vi "Enqueue - Multiple Commands.vi"(5 "Insert? (T)":bool=TRUE, 7 "At Front?":bool, 8 "error in":errorcluster, 10 "Array of Commands":string[](array[string]), 11 "Queue with Cluster Reference":T1) -> (0 "error out":errorcluster, 3 "Queue (dup)":T1)   [LabVIEW 2010]
uses:
  TYP_Queue with Cluster Reference.ctl
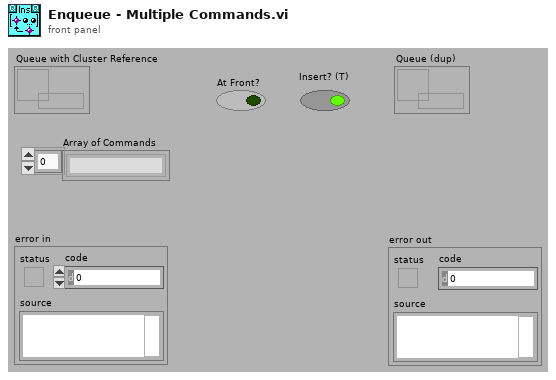
[diagram p1: front panel]
types:
  T1 = typedef "TYP_Queue with Cluster Reference.ctl" = refnum<queue>
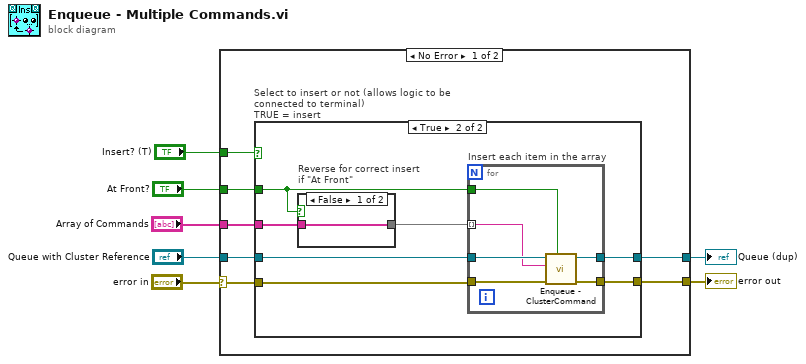
[diagram p0: block diagram]
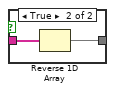
[diagram p3: hidden frame]
diagram:
  n1 = case shown="No Error" "error in" {
    selector: "error in" -> [w10 w34]
    tunnel: "Array of Commands" -> [w14 _]
    tunnel: "Queue with Cluster Reference" -> [w13 w33]
    tunnel: [w12 w33] -> w3
    tunnel: [w11 w34] -> w6
    tunnel: "At Front?" -> [w9 _]
    tunnel: "Insert? (T)" -> [w8 _]
    frame No Error {
      n2 = case "Select to insert or not (allows logic to be connected to terminal)\nTRUE = insert" shown="True" w8 {
        tunnel: w14 -> [_ w19]
        tunnel: w13 -> [w16 w23]
        tunnel: [w16 w22] -> w12
        tunnel: [w15 w21] -> w11
        tunnel: w10 -> [w15 w20]
        tunnel: w9 -> [_ w18]
        frame False {
        }
        frame True {
          n3 = case "Reverse for correct insert\nif \"At Front\"" shown="False" w18 {
            tunnel: w19 -> [w24 w26]
            tunnel: [w24 w25] -> w17
            frame False {
            }
            frame True {
              n4 = Reverse 1D Array(array=w26) -> (reversed array=w25:string[])
            }
          }
          n5 = for "Insert each item in the array" {
            tunnel: w23 -> [w29]
            tunnel: w20 -> [w32]
            tunnel: [w30] -> w22
            tunnel: [w31] -> w21
            tunnel: w17 -> [w28] mode=indexing
            tunnel: w18 -> [w27]
            n6 = call "Enqueue - ClusterCommand.vi"("At Front?"=w27, "error in (no error)"=w32, "Command"=w28, "Queue with Cluster Reference"=w29) -> ("error out"=w31:errorcluster, "Queue Out (dup)"=w30:T1)  [unwired: 6 in]
          }
        }
      }
    }
    frame Error {
    }
  }
  "error out" <- w6
  "Queue (dup)" <- w3
